vi "SaveIMAQImage.vi"(0 "IMAQ Image":T1) -> ()   [LabVIEW 2009]
uses:
  <vilib>/vision/Image Controls.llb/IMAQ Image.ctl
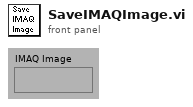
[diagram p1: front panel]
types:
  T1 = typedef "IMAQ Image.ctl" = refnum<image>
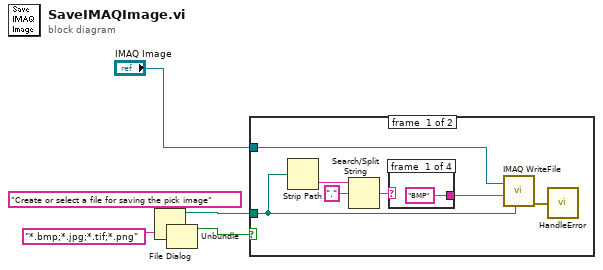
[diagram p0: block diagram]
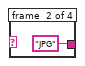
[diagram p2: hidden frame]
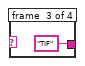
[diagram p3: hidden frame]
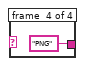
[diagram p4: hidden frame]
diagram:
  n1 = File Dialog(6:"*.bmp;*.jpg;*.tif;*.png" ("pattern"), 7:"Create or select a file for saving the pick image" ("prompt")) -> (0:w1:errorcluster, 1:w5:bool, 3:w4:path)  [unwired: 5 in, 1 out]
  n2 = Unbundle(w1) -> ()  [unwired: 3 out]
  n3 = case shown="False" w5 {
    tunnel: w4 -> [w13 _]
    tunnel: "IMAQ Image" -> [w7 _]
    frame #0 {
      n4 = Strip Path(path=w13) -> (name=w12:string)  [unwired: 1 out]
      n5 = Search/Split String(string=w12, search string/char (-)=".") -> (match + rest of string=w10:string)  [unwired: 1 in, 2 out]
      n6 = case shown="\".png\"" w10 {
        tunnel: ["BMP" ("File Type") "JPG" ("File Type") "TIF" ("File Type") "PNG" ("File Type")] -> w9
        frame #0 {
        }
        frame #1 {
        }
        frame #2 {
        }
        frame #3 {
        }
      }
      n7 = call "IMAQ WriteFile"("File Type"=w9, "File Path"=w13, "Image"=w7) -> ("error out"=w8:errorcluster)  [unwired: 5 in]
      n8 = call "HandleError.vi"("error in (no error)"=w8) -> ()
    }
    frame #1 {
    }
  }
